vi "csv_separador.vi"(5 "Archivo de referencias (.csv)":path) -> ()   [LabVIEW 2017]
panel:
  out "subarray 2":string[][](array[string])
  out "all rows":string[][](array[string])
  out "subarray":string[][](array[string])
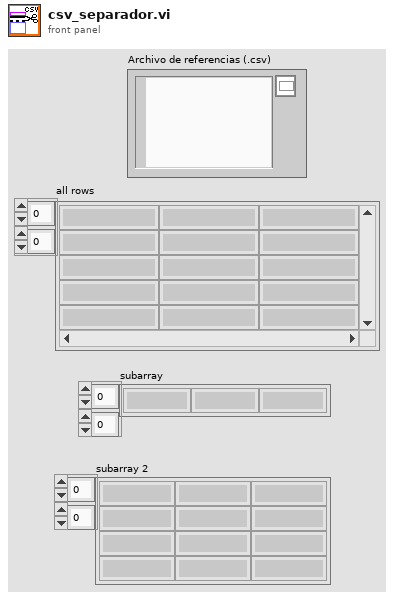
[diagram p1: front panel]
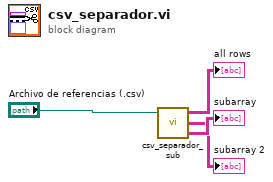
[diagram p0: block diagram]
diagram:
  n1 = call "csv_separador_sub.vi"("Archivo de referencias (.csv)"="Archivo de referencias (.csv)") -> ("subarray 2"=→"subarray":string[][], "subarray"=→"subarray 2":string[][], "all rows"=→"all rows":string[][])  [unwired: 2 in]
